vi "get Pmu Real Data Labview.vi"(0 "rd":cluster{"frequency":sgl, "deltaFrequency":sgl}, 1 "status":cluster{}, 2 "PhasorArrayLength":u16, 3 "phasorValueReal":sgl, 4 "phasorValueImaginary":sgl, 5 "AnalogArrayLength":u16, 6 "analogValueArr":sgl, 8 "DigitalArrayLength":u16, 9 "digitalValueArr":string, 10 "pseudoPdcId":i32, 11 "pmuIndex":i32) -> (19 "digitalValueArr out":string, 20 "rd out":cluster{"frequency":sgl, "deltaFrequency":sgl}, 21 "status out":cluster{}, 22 "function return":i32, 23 "phasorValueReal out":sgl, 24 "phasorValueImaginary out":sgl, 26 "analogValueArr out":sgl)   [LabVIEW 2012, in "C37118-DLL.lvlib" / "StrongridDLL.lvlib"]
doc: "STRONGRIDIEEEC37118DLL_API int __cdecl getPmuRealDataLabview(noArraysPmuDataFrame* rd, PmuStatus* status,\n uint16_t PhasorArrayLength, float* phasorValueReal, float* phasorValueImaginary,\n uint16_t AnalogArrayLength, float* analogValueArr,\n uint16_t DigitalArrayLength, uint8_t* digitalValueArr,\n int32_t pseudoPdcId, int32_t pmuIndex);"
uses:
  StrongridDLL.lvlib
  StrongridDLL.dll
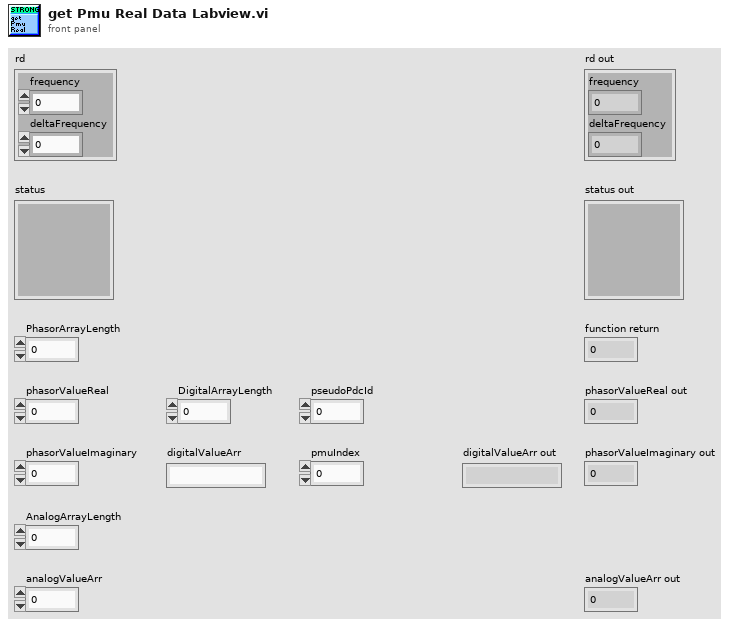
[diagram p1: front panel]
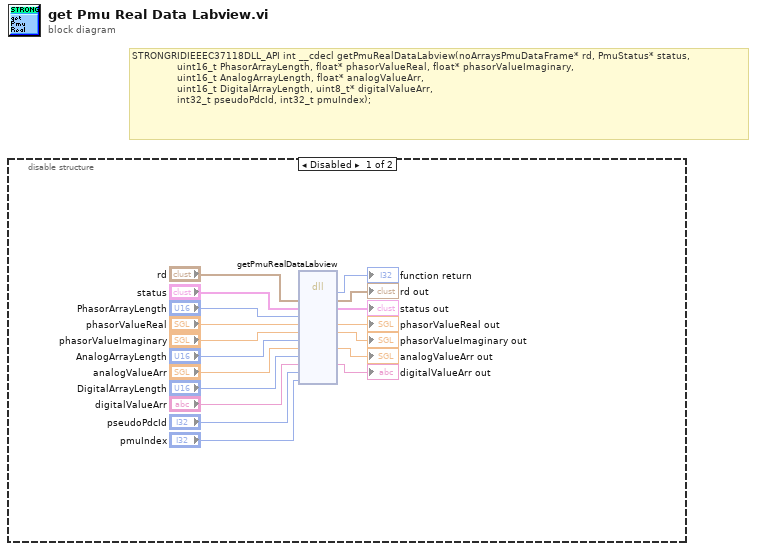
[diagram p0: block diagram]
diagram:
  # "STRONGRIDIEEEC37118DLL_API int __cdecl getPmuRealDataLabview(noArraysPmuDataFrame* rd, PmuStatus* status,\n\t\t\t\t\t\t\t\t\t\t\t\t\t\t\tuint16_t PhasorArrayLength, float* phasorValueReal, float* phasorValueImaginary,\n\t\t\t\t\t\t\t\t\t\t\t\t\t\t\tuint16_t AnalogArrayLength, float* analogValueArr,\n\t\t\t\t\t\t\t\t\t\t\t\t\t\t\tuint16_t DigitalArrayLength, uint8_t* digitalValueArr,\n\t\t\t\t\t\t\t\t\t\t\t\t\t\t\tint32_t pseudoPdcId, int32_t pmuIndex);"
  n1 = disable-structure shown="Disabled" {
    frame Disabled {
      n2 = dll-call lib="C:/__TSD-SVN/AFS171 Statnett License PMU Reference Library/source/LabVIEW PRL Library/c37118-dll/labview/vi/Auto Generated/StrongridDLL.*" fn="getPmuRealDataLabview"("rd"="rd", "status"="status", "PhasorArrayLength"="PhasorArrayLength", "phasorValueReal"="phasorValueReal", "phasorValueImaginary"="phasorValueImaginary", "AnalogArrayLength"="AnalogArrayLength", "analogValueArr"="analogValueArr", "DigitalArrayLength"="DigitalArrayLength", "digitalValueArr"="digitalValueArr", "pseudoPdcId"="pseudoPdcId", "pmuIndex"="pmuIndex") -> (→"function return":i32, "rd"=→"rd out":cluster{"frequency":sgl, "deltaFrequency":sgl}, "status"=→"status out":cluster{}, "phasorValueReal"=→"phasorValueReal out":sgl, "phasorValueImaginary"=→"phasorValueImaginary out":sgl, "analogValueArr"=→"analogValueArr out":sgl, "digitalValueArr"=→"digitalValueArr out":string)  [unwired: 8 in, 2 out]
    }
    frame Enabled {
    }
  }
